vi "appendXMLPoint.vi"(6 "error in (no error)":errorcluster, 7 "y":dbl, 8 "x":dbl, 9 "Parent Node":refnum<k20>, 10 "DOM document in":refnum<k20>) -> (0 "error out":errorcluster, 2 "Parent Node Out":refnum<k20>)   [LabVIEW 2013]
uses:
  <resource>/objmgr/DOMUserDefRef.rc
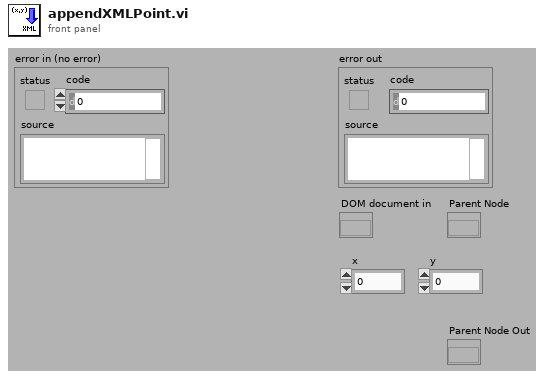
[diagram p1: front panel]
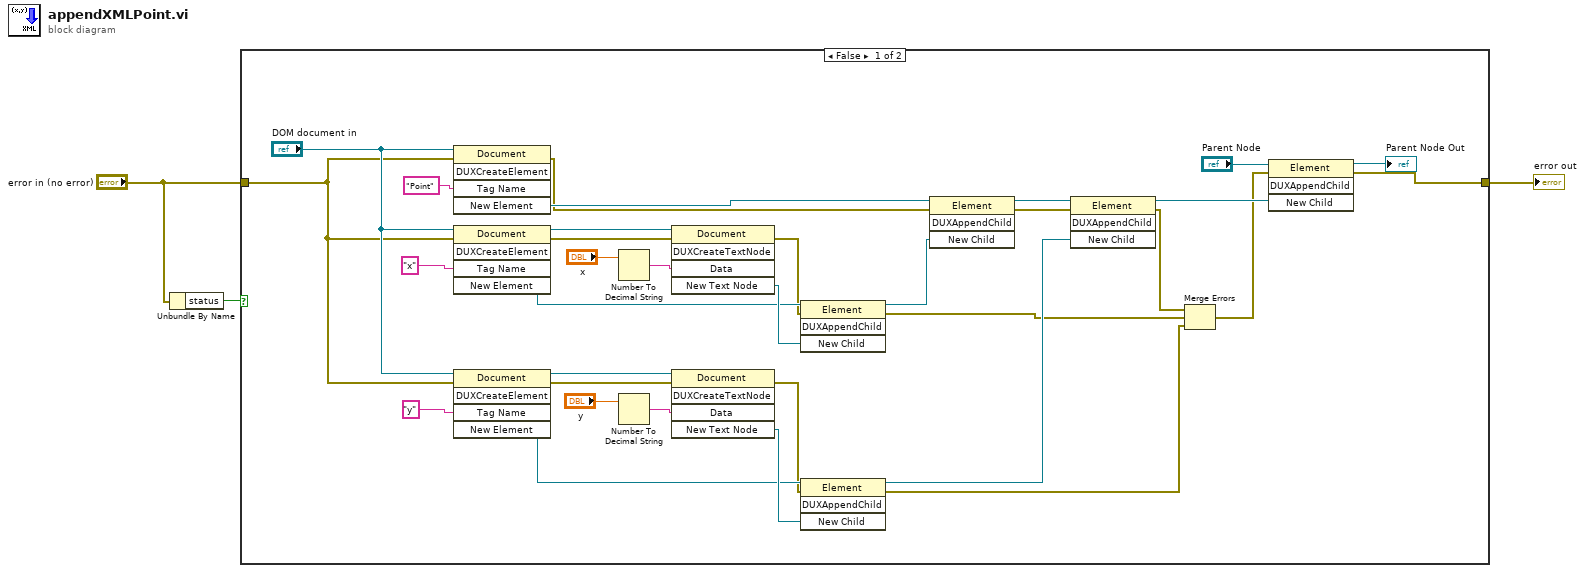
[diagram p0: block diagram]
diagram:
  n1 = Unbundle By Name("error in (no error)") -> ("status"=w2:bool)
  n2 = case shown="False" w2 {
    tunnel: "error in (no error)" -> [w5 w37]
    tunnel: [w4 w37] -> w3
    frame False {
      n3 = invoke class="Document" method="DUXCreateElement"(reference="DOM document in", error in=w5, "Tag Name"="Point") -> (error out=w14:errorcluster, "New Element"=w26:refnum<k20>)  [unwired: 2 in, 3 out]
      n4 = invoke class="Document" method="DUXCreateElement"(reference="DOM document in", error in=w5, "Tag Name"="x") -> (reference out=w25:refnum<k20>, error out=w15:errorcluster, "New Element"=w19:refnum<k20>)  [unwired: 2 in, 2 out]
      n5 = invoke class="Document" method="DUXCreateElement"(reference="DOM document in", error in=w5, "Tag Name"="y") -> (reference out=w32:refnum<k20>, error out=w11:errorcluster, "New Element"=w21:refnum<k20>)  [unwired: 2 in, 2 out]
      n6 = Number To Decimal String(number="x") -> (decimal integer string=w30:string)  [unwired: 1 in]
      n7 = Number To Decimal String(number="y") -> (decimal integer string=w28:string)  [unwired: 1 in]
      n8 = invoke class="Document" method="DUXCreateTextNode"(reference=w25, error in=w15, "Data"=w30) -> (error out=w12:errorcluster, "New Text Node"=w20:refnum<k20>)  [unwired: 2 in, 3 out]
      n9 = invoke class="Document" method="DUXCreateTextNode"(reference=w32, error in=w11, "Data"=w28) -> (error out=w10:errorcluster, "New Text Node"=w22:refnum<k20>)  [unwired: 2 in, 3 out]
      n10 = invoke class="Element" method="DUXAppendChild"(reference=w19, error in=w12, "New Child"=w20) -> (reference out=w18:refnum<k20>, error out=w9:errorcluster)  [unwired: 1 in, 2 out]
      n11 = invoke class="Element" method="DUXAppendChild"(reference=w21, error in=w10, "New Child"=w22) -> (reference out=w17:refnum<k20>, error out=w7:errorcluster)  [unwired: 1 in, 2 out]
      n12 = invoke class="Element" method="DUXAppendChild"(reference=w26, error in=w14, "New Child"=w18) -> (reference out=w27:refnum<k20>, error out=w13:errorcluster)  [unwired: 1 in, 2 out]
      n13 = invoke class="Element" method="DUXAppendChild"(reference=w27, error in=w13, "New Child"=w17) -> (reference out=w23:refnum<k20>, error out=w8:errorcluster)  [unwired: 1 in, 2 out]
      n14 = Merge Errors(w8, w9, w7) -> (w6:errorcluster)
      n15 = invoke class="Element" method="DUXAppendChild"(reference="Parent Node", error in=w6, "New Child"=w23) -> (reference out=→"Parent Node Out":refnum<k20>, error out=w4:errorcluster)  [unwired: 1 in, 2 out]
    }
    frame True {
    }
  }
  "error out" <- w3
